vi "Init Model.vi"(8 "error in":errorcluster, 11 "Notifiers in":T1) -> (0 "error out":errorcluster, 3 "Notifiers out":T1)   [LabVIEW 2015, in "Model.lvlib"]
uses:
  Model.lvlib
  support/Message Queue/Message Queue.lvlib
  support/Message Queue/Enqueue Message (Single).vi
  PLC/PLC.lvlib
  support/Notifiers/Notifiers.ctl
  support/Notifiers/Notifiers.lvlib
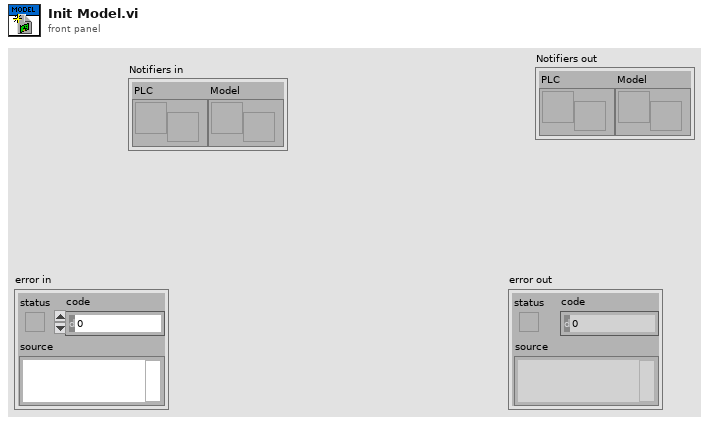
[diagram p1: front panel]
types:
  T1 = typedef "Notifiers.lvlib/Notifiers.ctl" = cluster{"PLC":refnum<notifier>, "Model":refnum<notifier>}
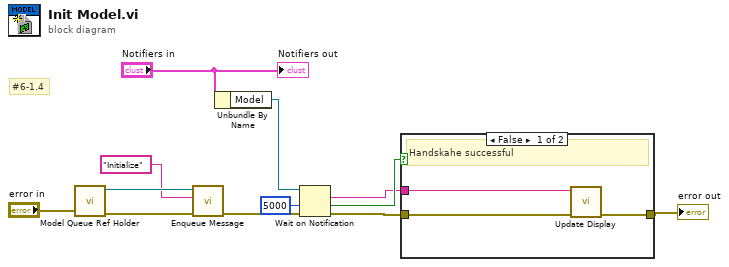
[diagram p0: block diagram]
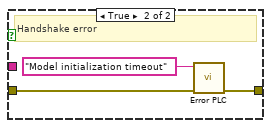
[diagram p2: hidden frame]
diagram:
  # "#6-1.4"
  n1 = call "Model Queue Ref Holder.vi"("error in"="error in") -> ("error out"=w8:errorcluster, "Input Message Queue"=w7:refnum<queue>)  [unwired: 9 in]
  n2 = call-poly "Enqueue Message.vi"("error in (no error)"=w8, "Message"="Initialize", "Message Queue"=w7) -> ("error out"=w10:errorcluster)  [unwired: 7 in, 1 out]
  n3 = Unbundle By Name("Notifiers in") -> ("Model"=w1:refnum<notifier>)
  n4 = Wait on Notification(notifier=w1, timeout in ms (-1)=5000, error in (no error)=w10) -> (notification=w9:string, timed out?=w11:bool, error out=w12:errorcluster)  [unwired: 1 in, 1 out]
  n5 = case shown="False" w11 {
    tunnel: w12 -> [w15 w17]
    tunnel: [w14 w16] -> w6
    tunnel: w9 -> [w13 _]
    frame False {
      # "Handskahe successful"
      n6 = call "Update Display.vi"("error in"=w15, "Message string"=w13) -> ("error out"=w14:errorcluster)  [unwired: 9 in]
    }
    frame True {
      # "Handshake error"
      n7 = call "Error PLC.vi"("error in"=w17, "String"="Model initialization timeout" ("Message")) -> ("error out"=w16:errorcluster)  [unwired: 9 in]
    }
  }
  "error out" <- w6
  "Notifiers out" <- "Notifiers in"
